vi "NIVS PWM In.vi"(2 "PWM In Timeout":u32, 3 "DI":bool) -> (0 "PWM In Freq Packet":u64, 1 "PWM In DC Packet":u64)   [LabVIEW 2014]
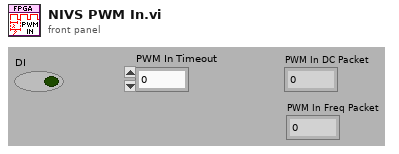
[diagram p1: front panel]
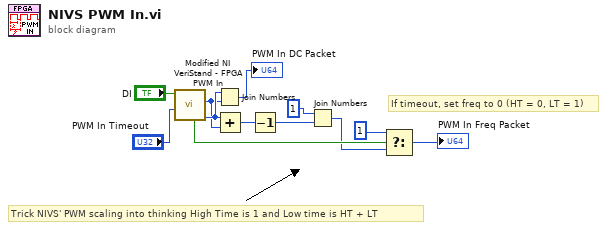
[diagram p0: block diagram]
diagram:
  # "If timeout, set freq to 0 (HT = 0, LT = 1)"
  # "Trick NIVS' PWM scaling into thinking High Time is 1 and Low time is HT + LT"
  n1 = call "Modified NI VeriStand - FPGA PWM In.vi"("Time Out"="PWM In Timeout", "Value"="DI") -> ("High time"=w12:u32, "Low Time"=w11:u32, "Timeout?"=w6:bool)  [unwired: 7 out]
  n2 = Join Numbers(hi=w12, lo=w11) -> ((hi.lo)=→"PWM In DC Packet":u64)
  n3 = Add(x=w12, y=w11) -> (x+y=w8:u32)
  n4 = Decrement(x=w8) -> (x-1=w7:u32)
  n5 = Join Numbers(hi=u32 1, lo=w7) -> ((hi.lo)=w4:u64)
  n6 = Select(t=u64 1 ("(hi.lo)"), s=w6, f=w4) -> (s? t:f=→"PWM In Freq Packet":u64)
